vi "Helm Send All Stop.vi"(8 "error in (no error)":errorcluster) -> (0 "error out":errorcluster, 3 "All Stop Message":refnum<class "Steering Command.lvclass">)   [LabVIEW 2015, in "RDS Helm Actor.lvlib"]
uses:
  RDS Helm Actor.lvlib
  Libraries/RDS Child Messages/Helm/Steering Command/Steering Command.lvclass
  Libraries/RDS Framework/RDS Message ID.ctl
  Libraries/RDS Child Messages/Helm/Steering Command/Steering Command Cntrl.ctl
  Libraries/RDS Framework/RDS Message Class/RDS Message.lvclass/RDS Message.ctl
  Libraries/RDS Child Messages/Helm/Steering Command/Steering Command.lvclass/Steering Command.ctl
  Libraries/RDS Framework/RDS Message Class/RDS Message.lvclass
  Libraries/RDS Child Messages/RDS Child Messages.lvlib
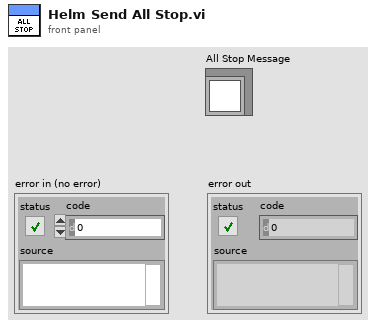
[diagram p1: front panel]
types:
  T1 = typedef "RDS Child Messages.lvlib/Steering Command Cntrl.ctl" = cluster{"Throttle":i16, "Rudder":i8, "Duration (s)":u16}
  T2 = typedef "RDS Child Messages.lvlib/RDS Message ID.ctl" = enum16{"RDS Hello World", "String Message", "AIP_Status", "AIP_Command", "GPS_Data", "MCB_Command", "MCB_Status", "Compass_Data", "Depth_Data", "Battery_Data", "Contoller_State", "Set_Mag_Dev", "BTB_Shutdown", "State_Sample_Request", "State_Sample", "PID_Gains_Set", "Helm_Limiter_Set", "Helm_Heading_Command", "Helm_Steering_Command", "Helm_Status", "Controller_Message", "AIP_Set_Min_Depth", "Mission_Controller_State", "Mission_Upload", "Mission_Set_Op_and_Run", "Mission_Settings_Set"}
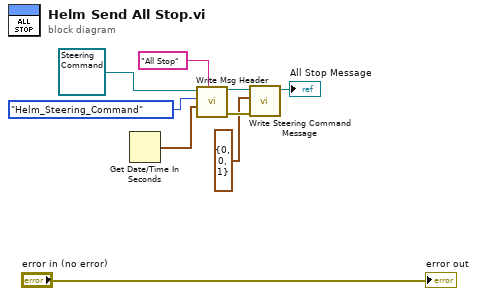
[diagram p0: block diagram]
diagram:
  n1 = Get Date/Time In Seconds() -> (seconds since 1Jan1904=w3:timestamp)
  n2 = call "Write Msg Header.vi"("Sender Name"="All Stop", "Time Stamp"=w3, "Msg ID"=RDS_Message_ID."Helm_Steering_Command", "RDS Message in"=refnum<class "Steering Command.lvclass"> refnum ("RDS Child Messages.lvlib:Steering Command.lvclass")) -> ("error out"=w9:errorcluster, "RDS Message out"=w7:refnum<class "Steering Command.lvclass">)  [unwired: 6 in]
  n3 = call "Write Steering Command Message.vi"("error in (no error)"=w9, "Steering Command Control"=T1 {"Throttle"=0, "Rudder"=0, "Duration (s)"=1}, "Steering Command in"=w7) -> ("Steering Command out"=→"All Stop Message":refnum<class "Steering Command.lvclass">)  [unwired: 7 in, 1 out]
  "error out" <- "error in (no error)"
